vi "MultiBallAuton.vi"() -> ()   [LabVIEW 2014]
uses:
  TwoBallAuton.ctl
  Events.vi
panel:
  out "State":T1(ring)=enum."GetBall"
  out "GrabCount":i32
  # "Variables"
  # "Outputs"
  # "Inputs"
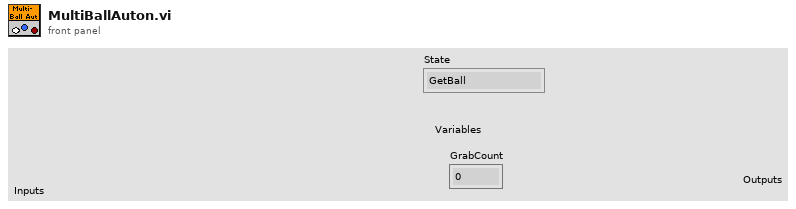
[diagram p1: front panel]
types:
  T1 = enum16{"Start", "LineUp", "Fire", "Reload", "GetBall", "Finish"}
  T2 = typedef "TwoBallAuton.ctl" = enum16{"Start", "LineUp", "Fire", "Reload", "GetBall", "Finish"}
  T3 = typedef "Eventgrab.ctl" = cluster{"Grab":bool, "GroundPass":bool, "Test Aqaure":dbl, "Shoulder up or down?":bool, "Auton drag":bool}
  T4 = cluster{"Translate":dbl, "Y-Axis (Backward Speed)":dbl, "Rotate":dbl, "Tank right side":dbl, "axis 5":dbl, "axis 6":dbl, "Use gyro":bool, "Exponential\ndrive":bool, "Ring light":bool, "PID rotation":bool, "PID Gain":dbl}
  T5 = cluster{"Reloading?":bool, "Throw":bool, "Ready?":bool, "Truss throw":bool, "Power is high?":bool, "Automatic relaod?":bool, "Manuall servo":bool}
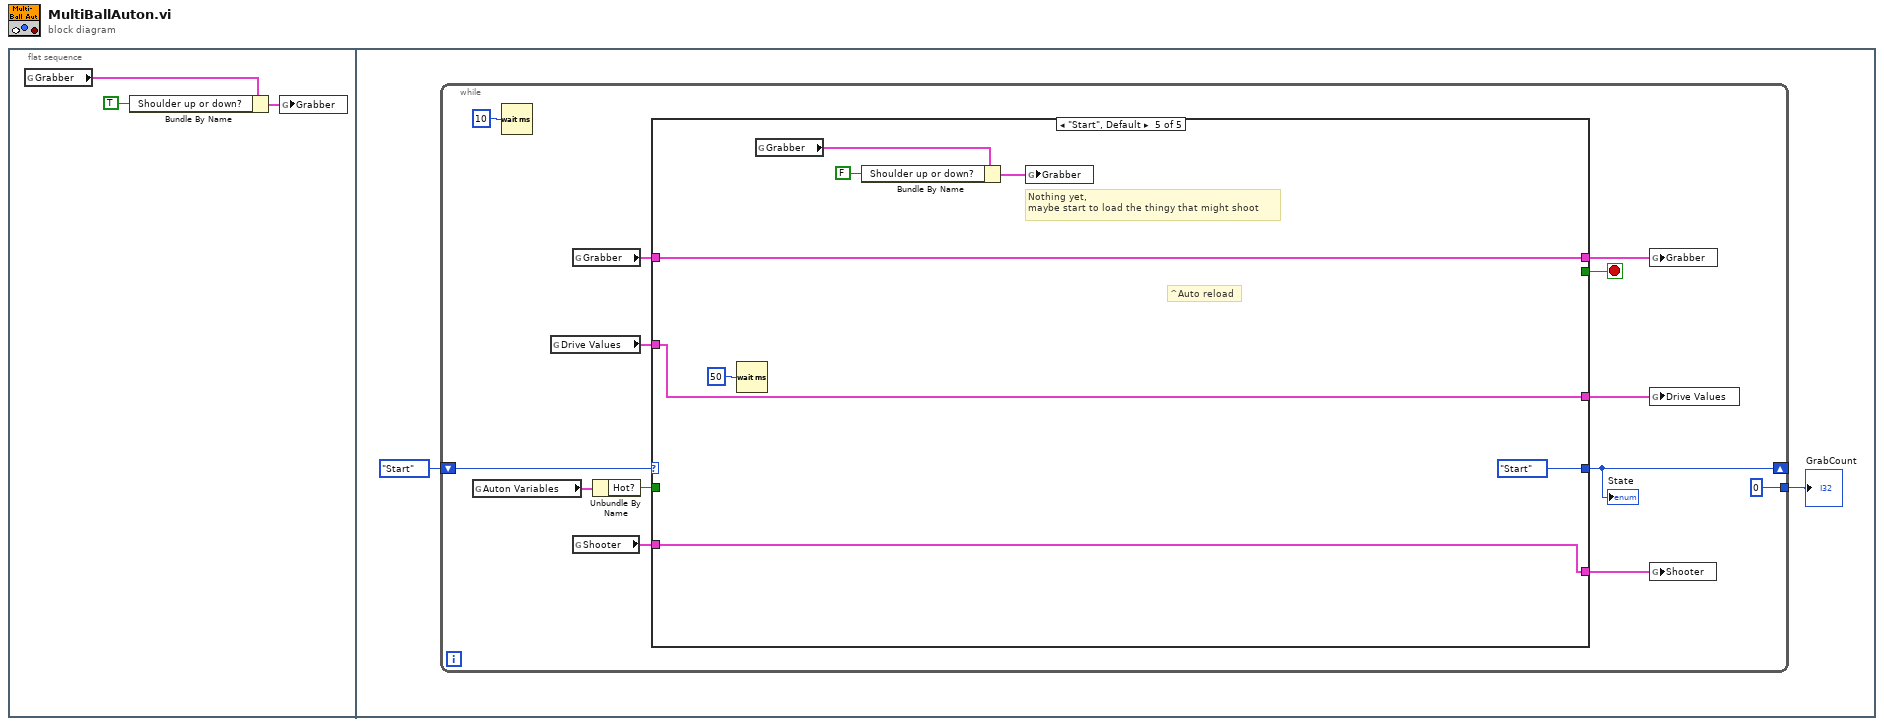
[diagram p0: block diagram]
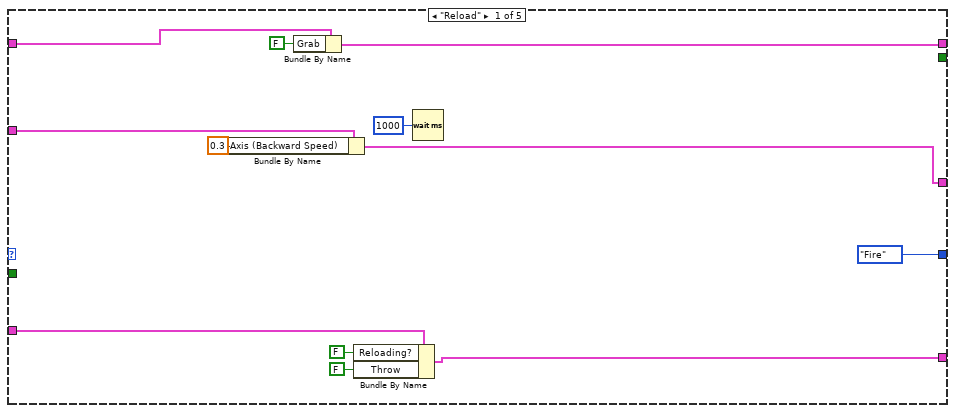
[diagram p2: hidden frame]
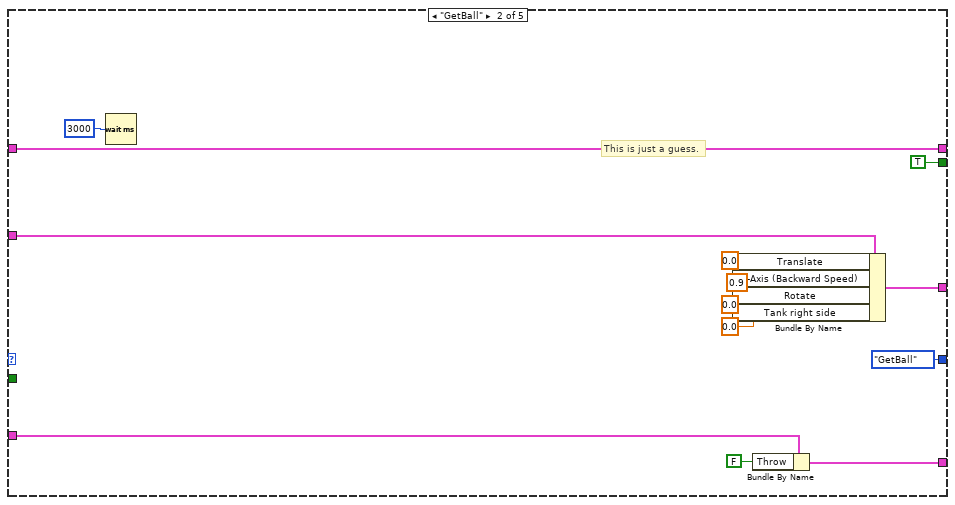
[diagram p3: hidden frame]
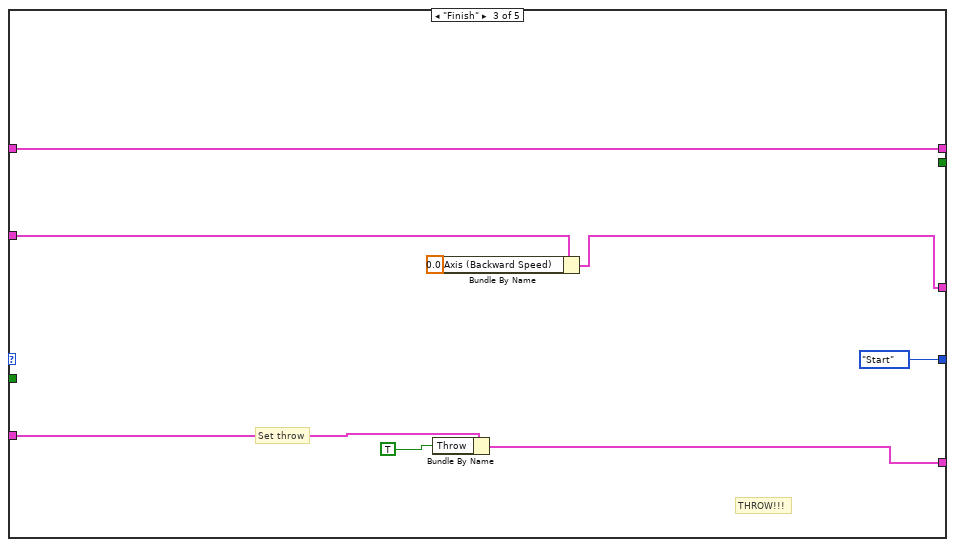
[diagram p4: hidden frame]
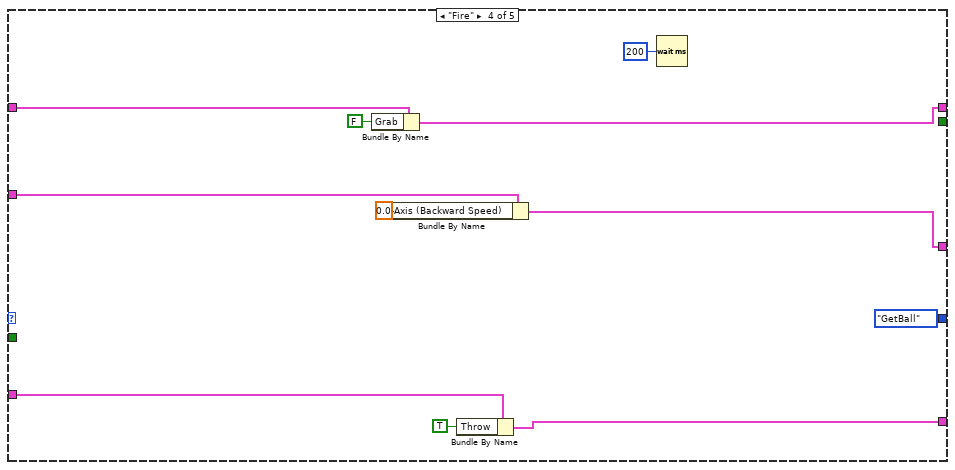
[diagram p5: hidden frame]
diagram:
  n1 = flat-sequence {
    frame #0 {
      n2 = global read "Events.vi" "Grabber"() -> (w2:T3)
      n3 = Bundle By Name(cluster=w2, "Shoulder up or down?"=TRUE) -> (w3:T3)
      n4 = global write "Events.vi" "Grabber"(w3) -> ()
    }
    frame #1 {
      n5 = while {
        shift-right: [w17] -> _
        shift-left: TwoBallAuton."Start" -> [w6]
        tunnel: [0] -> w4
        stop <- w7 stop-if-true
        n6 = global read "Events.vi" "Auton Variables"() -> (w12:cluster{"Hot?":bool, "WhichAuton":string})
        n7 = Wait (ms)(milliseconds to wait=u32 10) -> ()  [unwired: 1 out]
        n8 = global read "Events.vi" "Drive Values"() -> (w14:T4)
        n9 = global read "Events.vi" "Grabber"() -> (w13:T3)
        n10 = global read "Events.vi" "Shooter"() -> (w15:T5)
        n11 = Unbundle By Name(w12) -> ("Hot?"=w11:bool)
        n12 = case shown="\"Start\", Default" w6 {
          tunnel: [TwoBallAuton."Fire" TwoBallAuton."GetBall" TwoBallAuton."Start" TwoBallAuton."GetBall" TwoBallAuton."Start"] -> w17
          tunnel: [_ TRUE _ _ _] -> w7
          tunnel: w11 -> [_ _ _ _ _]
          tunnel: w15 -> [w23 w33 w49 w62 w68]
          tunnel: w14 -> [w30 w36 w47 w59 w70]
          tunnel: w13 -> [w26 w41 w51 w56 w69]
          tunnel: [w29 w35 w46 w58 w70] -> w10
          tunnel: [w25 w41 w51 w55 w69] -> w9
          tunnel: [w22 w32 w48 w61 w68] -> w8
          frame "Reload" {
            n13 = Bundle By Name(cluster=w30, "Y-Axis (Backward Speed)"=0.3 ("Forward Speed")) -> (w29:T4)
            n14 = Bundle By Name(cluster=w26, "Grab"=FALSE) -> (w25:T3)
            n15 = Bundle By Name(cluster=w23, "Reloading?"=FALSE, "Throw"=FALSE) -> (w22:T5)
            n16 = Wait (ms)(milliseconds to wait=u32 1000) -> ()  [unwired: 1 out]
          }
          frame "GetBall" {
            # "This is just a guess."
            n17 = Wait (ms)(milliseconds to wait=u32 3000) -> ()  [unwired: 1 out]
            n18 = Bundle By Name(cluster=w36, "Translate"=0.0, "Y-Axis (Backward Speed)"=0.9 ("Forward Speed"), "Rotate"=0.0, "Tank right side"=0.0) -> (w35:T4)
            n19 = Bundle By Name(cluster=w33, "Throw"=FALSE) -> (w32:T5)
          }
          frame "Finish" {
            # "Set throw"
            # "THROW!!!"
            n20 = Bundle By Name(cluster=w47, "Y-Axis (Backward Speed)"=0.0 ("Forward Speed")) -> (w46:T4)
            n21 = Bundle By Name(cluster=w49, "Throw"=TRUE) -> (w48:T5)
          }
          frame "Fire" {
            n22 = Bundle By Name(cluster=w56, "Grab"=FALSE) -> (w55:T3)
            n23 = Bundle By Name(cluster=w59, "Y-Axis (Backward Speed)"=0.0 ("Forward Speed")) -> (w58:T4)
            n24 = Bundle By Name(cluster=w62, "Throw"=TRUE) -> (w61:T5)
            n25 = Wait (ms)(milliseconds to wait=u32 200) -> ()  [unwired: 1 out]
          }
          frame "Start", Default {
            # "^Auto reload"
            # "Nothing yet,\nmaybe start to load the thingy that might shoot"
            n26 = Wait (ms)(milliseconds to wait=u32 50) -> ()  [unwired: 1 out]
            n27 = global read "Events.vi" "Grabber"() -> (w65:T3)
            n28 = Bundle By Name(cluster=w65, "Shoulder up or down?"=FALSE) -> (w66:T3)
            n29 = global write "Events.vi" "Grabber"(w66) -> ()
          }
        }
        "State" <- w17
        n30 = global write "Events.vi" "Grabber"(w9) -> ()
        n31 = global write "Events.vi" "Drive Values"(w10) -> ()
        n32 = global write "Events.vi" "Shooter"(w8) -> ()
      }
      "GrabCount" <- w4
    }
  }
